vi "ESC_Send value.vi"(3 "Error In":errorcluster, 4 "Output (0...1)":sgl, 5 "Port":refnum<visa-resource-name>) -> (0 "Error Out":errorcluster, 1 "Output":sgl, 2 "Port out":refnum<visa-resource-name>)   [LabVIEW 2020]
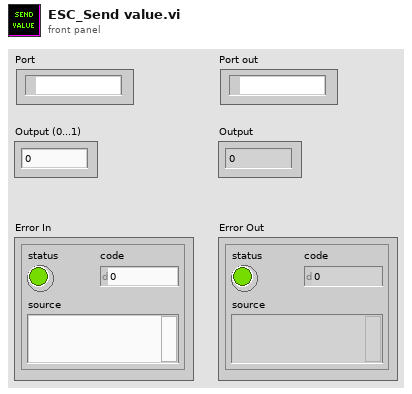
[diagram p1: front panel]
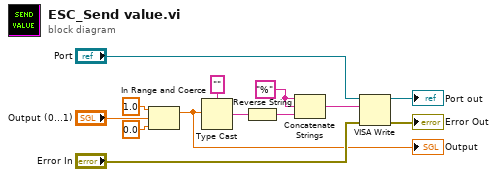
[diagram p0: block diagram]
diagram:
  w5 = "%"
  n1 = In Range and Coerce(upper limit=sgl 1.0, x="Output (0...1)", lower limit=sgl 0.0) -> (coerced(x)=w1:sgl)  [unwired: 1 out]
  "Output" <- w1
  n2 = Type Cast(type="", x=w1) -> (*(type *) &x=w12:string)
  n3 = Reverse String(1:w12) -> (0:w11:string)
  n4 = Concatenate Strings(w5, w5, w11) -> (w10:string)
  n5 = VISA Write(VISA resource name="Port", write buffer=w10, error in (no error)="Error In") -> (VISA resource name out=→"Port out":refnum<visa-resource-name>, error out=→"Error Out":errorcluster)  [unwired: 1 out]
